vi "Measure.vi"(8 "error in":errorcluster, 10 "Controle":T1, 11 "map reference in":refnum<data-value>) -> (0 "error out":errorcluster, 2 "Indicator":T1, 3 "map reference out":refnum<data-value>, 4 "Occupancy Grid":dbl[][](graph), 6 "XY Graph":cluster{dbl[], dbl[]}[](graph))   [LabVIEW 2011]
uses:
  <vilib>/robotics/Navigation/shared/WorldMap/OccupancyGridWorldMap/NI_Robotics_OccupancyGridWorldMap.lvclass
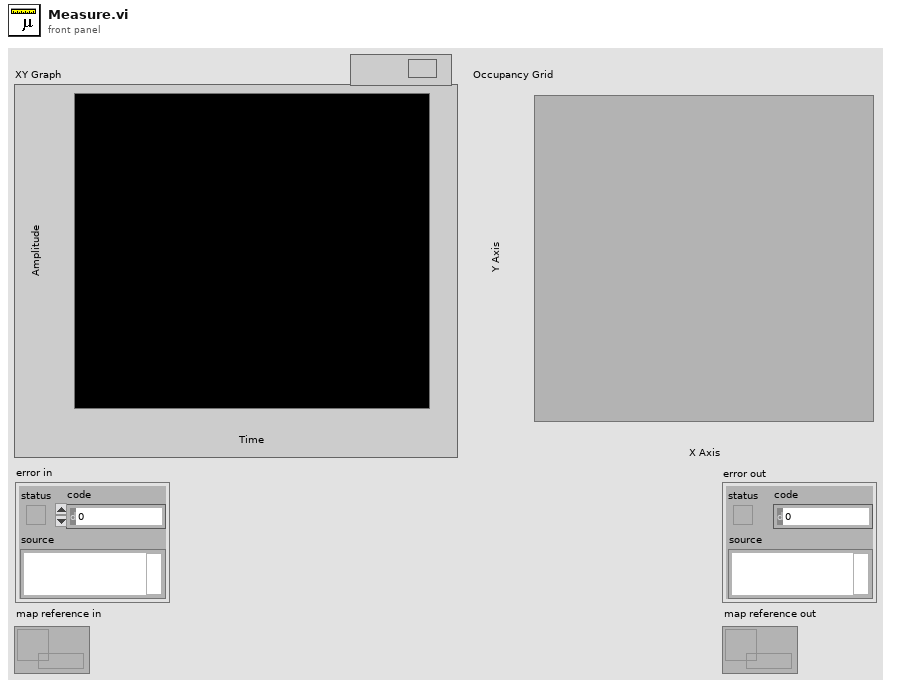
[diagram p1: front panel]
types:
  T1 = cluster{"Resolution":i32, "Scale":dbl, "Data":cluster{"GPS Data":cluster{"Latitude":dbl, "Longitude":dbl, "Altitude":dbl, "Velocity, Correction & SET":cluster{"Velocity North":dbl, "Velocity East":dbl, "Velocity Up":dbl, "Ellipsoidal Height":dbl, "GDOP":sgl, "PDOP":sgl, "HDOP":sgl, "VDOP":sgl, "TDOP":sgl, "Horizontal Figure of Merit":u8, "Time Figure of Merit":u8, "Max dGPS Age":sgl, "Extended Navigation Mode":u8, "Antenna Height Adjustment ":dbl, "SET North":i32, "SET East":i32, "SET Up":i32}, "Time":cluster{"GPS Week":u16, "GPS Time of Week":sgl}, "Satellites Used":i32[]}, "IMU Data":cluster{"Position":cluster{"Roll":dbl, "Pitch":dbl, "Yaw":dbl}, "Orientation Matrix":dbl[][], "Magnetic Field":cluster{"Z-Axis Magnetic Field":dbl, "Y-Axis Magnetic Field":dbl, "X-Axis Magnetic Field":dbl}, "Acceleration":cluster{"Z-Axis Acceleration":dbl, "Y-Axis Acceleration":dbl, "X-Axis Acceleration":dbl}, "Angular Rate":cluster{"X-Axis Angular Rate":dbl, "Y-Axis Angular Rate":dbl, "Z-Axis Angular Rate":dbl}, "Quaternion":dbl[]}, "LIDAR Data":cluster{"Magnitude":dbl[], "Direction":dbl[]}, "Telemetry":cluster{"Voltage":cluster{sgl, sgl, sgl}, "Encoder Speed":cluster{i32, i32}, "Temps":cluster{"IC Temp (C)":i32, "Ch1 Temp (C)":i32, "Ch2 Temp (C)":i32}, "Current":cluster{dbl, dbl, dbl, dbl}}, "Lines":cluster{"Start Point":cluster{"X":sgl, "Y":sgl}, "End Point":cluster{"X":sgl, "Y":sgl}, "Length":dbl, "Orientation":dbl, "Score":dbl}[]}, "initialized array":dbl[][]}
  T2 = cluster{"Voltage":cluster{sgl, sgl, sgl}, "Encoder Speed":cluster{i32, i32}, "Temps":cluster{"IC Temp (C)":i32, "Ch1 Temp (C)":i32, "Ch2 Temp (C)":i32}, "Current":cluster{dbl, dbl, dbl, dbl}}
  T3 = cluster{"Latitude":dbl, "Longitude":dbl, "Altitude":dbl, "Velocity, Correction & SET":cluster{"Velocity North":dbl, "Velocity East":dbl, "Velocity Up":dbl, "Ellipsoidal Height":dbl, "GDOP":sgl, "PDOP":sgl, "HDOP":sgl, "VDOP":sgl, "TDOP":sgl, "Horizontal Figure of Merit":u8, "Time Figure of Merit":u8, "Max dGPS Age":sgl, "Extended Navigation Mode":u8, "Antenna Height Adjustment ":dbl, "SET North":i32, "SET East":i32, "SET Up":i32}, "Time":cluster{"GPS Week":u16, "GPS Time of Week":sgl}, "Satellites Used":i32[]}
  T4 = cluster{"Position":cluster{"Roll":dbl, "Pitch":dbl, "Yaw":dbl}, "Orientation Matrix":dbl[][], "Magnetic Field":cluster{"Z-Axis Magnetic Field":dbl, "Y-Axis Magnetic Field":dbl, "X-Axis Magnetic Field":dbl}, "Acceleration":cluster{"Z-Axis Acceleration":dbl, "Y-Axis Acceleration":dbl, "X-Axis Acceleration":dbl}, "Angular Rate":cluster{"X-Axis Angular Rate":dbl, "Y-Axis Angular Rate":dbl, "Z-Axis Angular Rate":dbl}, "Quaternion":dbl[]}
  T5 = cluster{"Start Point":cluster{"X":sgl, "Y":sgl}, "End Point":cluster{"X":sgl, "Y":sgl}, "Length":dbl, "Orientation":dbl, "Score":dbl}[]
  T6 = cluster{"GPS Data":cluster{"Latitude":dbl, "Longitude":dbl, "Altitude":dbl, "Velocity, Correction & SET":cluster{"Velocity North":dbl, "Velocity East":dbl, "Velocity Up":dbl, "Ellipsoidal Height":dbl, "GDOP":sgl, "PDOP":sgl, "HDOP":sgl, "VDOP":sgl, "TDOP":sgl, "Horizontal Figure of Merit":u8, "Time Figure of Merit":u8, "Max dGPS Age":sgl, "Extended Navigation Mode":u8, "Antenna Height Adjustment ":dbl, "SET North":i32, "SET East":i32, "SET Up":i32}, "Time":cluster{"GPS Week":u16, "GPS Time of Week":sgl}, "Satellites Used":i32[]}, "IMU Data":cluster{"Position":cluster{"Roll":dbl, "Pitch":dbl, "Yaw":dbl}, "Orientation Matrix":dbl[][], "Magnetic Field":cluster{"Z-Axis Magnetic Field":dbl, "Y-Axis Magnetic Field":dbl, "X-Axis Magnetic Field":dbl}, "Acceleration":cluster{"Z-Axis Acceleration":dbl, "Y-Axis Acceleration":dbl, "X-Axis Acceleration":dbl}, "Angular Rate":cluster{"X-Axis Angular Rate":dbl, "Y-Axis Angular Rate":dbl, "Z-Axis Angular Rate":dbl}, "Quaternion":dbl[]}, "LIDAR Data":cluster{"Magnitude":dbl[], "Direction":dbl[]}, "Telemetry":cluster{"Voltage":cluster{sgl, sgl, sgl}, "Encoder Speed":cluster{i32, i32}, "Temps":cluster{"IC Temp (C)":i32, "Ch1 Temp (C)":i32, "Ch2 Temp (C)":i32}, "Current":cluster{dbl, dbl, dbl, dbl}}, "Lines":cluster{"Start Point":cluster{"X":sgl, "Y":sgl}, "End Point":cluster{"X":sgl, "Y":sgl}, "Length":dbl, "Orientation":dbl, "Score":dbl}[]}
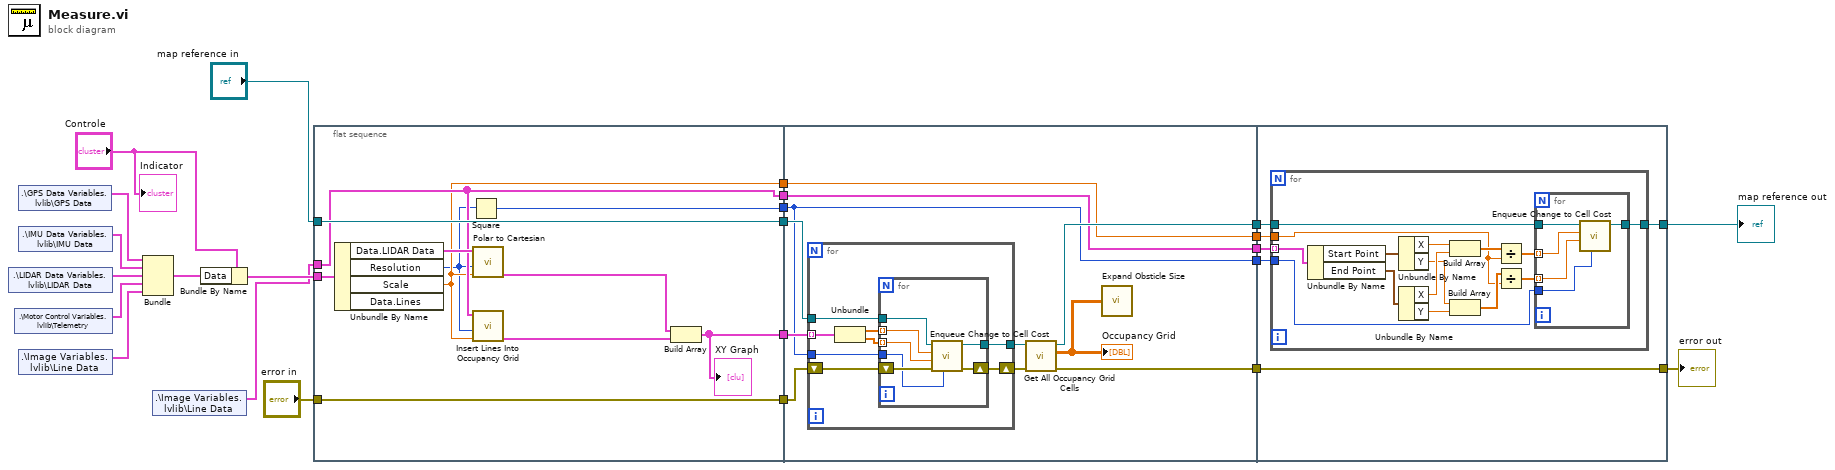
[diagram p0: block diagram]
diagram:
  n1 = shared-variable ".\\LIDAR Data Variables.lvlib\\LIDAR Data"() -> (w18:cluster{"Magnitude":dbl[], "Direction":dbl[]})  [unwired: 1 in, 1 out]
  n2 = shared-variable ".\\Motor Control Variables.lvlib\\Telemetry"() -> (w17:T2)  [unwired: 1 in, 1 out]
  n3 = shared-variable ".\\GPS Data Variables.lvlib\\GPS Data"() -> (w20:T3)  [unwired: 1 in, 1 out]
  n4 = shared-variable ".\\IMU Data Variables.lvlib\\IMU Data"() -> (w19:T4)  [unwired: 1 in, 1 out]
  n5 = shared-variable ".\\Image Variables.lvlib\\Line Data"() -> (w16:T5)  [unwired: 1 in, 1 out]
  n6 = Bundle("GPS Data"=w20, "IMU Data"=w19, "LIDAR Data"=w18, "Telemetry"=w17, "Lines"=w16) -> (w15:T6)  [unwired: 1 in]
  n7 = shared-variable ".\\Image Variables.lvlib\\Line Data"() -> (w12:T5)  [unwired: 1 in, 1 out]
  n8 = Bundle By Name(cluster="Controle", "Data"=w15) -> (w14:T1)
  n9 = flat-sequence {
    tunnel: "map reference in" -> [w35]
    tunnel: [w35] -> w21
    tunnel: w14 -> [w34]
    tunnel: w12 -> [w29]
    tunnel: [w30] -> w11
    tunnel: [w29] -> w7
    tunnel: [w28] -> w5
    tunnel: [w26] -> w4
    tunnel: "error in" -> [w25]
    tunnel: [w25] -> w1
    tunnel: w21 -> [w42]
    tunnel: w11 -> [w45]
    tunnel: [w44] -> w10
    tunnel: [w43] -> w9
    tunnel: [w39] -> w8
    tunnel: w7 -> [w39]
    tunnel: [w38] -> w6
    tunnel: w5 -> [w38]
    tunnel: w4 -> [w37]
    tunnel: [w37] -> w3
    tunnel: w1 -> [w36]
    tunnel: [w67] -> w23
    tunnel: [w63] -> w24
    tunnel: w10 -> [w64]
    tunnel: w9 -> [w67]
    tunnel: w8 -> [w66]
    tunnel: w6 -> [w65]
    tunnel: w3 -> [w62]
    frame #0 {
      n10 = Unbundle By Name(w34) -> ("Data.LIDAR Data"=w33:cluster{"Magnitude":dbl[], "Direction":dbl[]}, "Resolution"=w27:i32, "Scale"=w28:dbl)  [unwired: 1 out]
      n11 = Square(x=w27) -> (x^2=w26:i32)
      n12 = call "Polar to Cartesian.vi"("Scale"=w28, "Resulotion"=w27, "LIDAR Data"=w33) -> ("XY"=w32:cluster{dbl[], dbl[]})  [unwired: 7 in, 1 out]
      n13 = call "Insert Lines Into Occupancy Grid.vi"("Scale"=w28, "Resolution"=w27, "Lines In"=w29) -> ("XY"=w31:cluster{dbl[], dbl[]})  [unwired: 7 in, 1 out]
      n14 = Build Array(w32, w31) -> (w30:cluster{dbl[], dbl[]}[])
      "XY Graph" <- w30
    }
    frame #1 {
      n15 = for {
        tunnel: [w54] -> w46
        tunnel: w45 -> [w51] mode=indexing
        tunnel: w42 -> [w50]
        shift-right: [w48] -> w41
        shift-left: w36 -> [w49]
        tunnel: w37 -> [w47]
        n16 = Unbundle(w51) -> (w52:dbl[], w53:dbl[])
        n17 = for {
          tunnel: w52 -> [w60] mode=indexing
          tunnel: w53 -> [w61] mode=indexing
          tunnel: w50 -> [w59]
          tunnel: [w58] -> w54
          shift-right: [w56] -> w48
          shift-left: w49 -> [w57]
          tunnel: w47 -> [w55]
          n18 = call <vilib>:"Enqueue Change to Cell Cost.vi"("cost"=w55, "error in (no error)"=w57, "y"=w61, "x"=w60, "map reference in"=w59) -> ("error out"=w56:errorcluster, "map reference out"=w58:refnum<data-value>)  [unwired: 5 in]
        }
      }
      n19 = call <vilib>:"Get All Occupancy Grid Cells.vi"("error in (no error)"=w41, "map reference in"=w46) -> ("error out"=w43:errorcluster, "occupancy grid"=w40:dbl[][], "map reference out"=w44:refnum<data-value>)  [unwired: 7 in]
      "Occupancy Grid" <- w40
      n20 = call "Expand Obsticle Size.vi"("Map In"=w40) -> ()  [unwired: 1 out]
    }
    frame #2 {
      n21 = for {
        tunnel: w66 -> [w82] mode=indexing
        tunnel: w65 -> [w73]
        tunnel: w64 -> [w70]
        tunnel: [w69] -> w63
        tunnel: w62 -> [w68]
        n22 = Unbundle By Name(w82) -> ("Start Point"=w80:cluster{"X":sgl, "Y":sgl}, "End Point"=w81:cluster{"X":sgl, "Y":sgl})
        n23 = Unbundle By Name(w80) -> ("X"=w79:sgl, "Y"=w77:sgl)
        n24 = Unbundle By Name(w81) -> ("X"=w78:sgl, "Y"=w76:sgl)
        n25 = Build Array(w79, w78) -> (w75:sgl[])
        n26 = Build Array(w77, w76) -> (w74:sgl[])
        n27 = Divide(x=w75, y=w73) -> (x/y=w72:dbl[])
        n28 = Divide(x=w74, y=w73) -> (x/y=w71:dbl[])
        n29 = for {
          tunnel: w72 -> [w85] mode=indexing
          tunnel: w71 -> [w84] mode=indexing
          tunnel: w70 -> [w86]
          tunnel: [w87] -> w69
          tunnel: w68 -> [w83]
          n30 = call <vilib>:"Enqueue Change to Cell Cost.vi"("cost"=w83, "y"=w84, "x"=w85, "map reference in"=w86) -> ("map reference out"=w87:refnum<data-value>)  [unwired: 6 in, 1 out]
        }
      }
    }
  }
  "map reference out" <- w24
  "error out" <- w23
  "Indicator" <- "Controle"
